vi "Write.vi"(8 "error in (no error)":errorcluster, 10 "Bytes":u8[](array[numeric]) format="%08b", 11 "Connection in":refnum<class "Connection.lvclass">) -> (0 "error out":errorcluster, 3 "Connection":refnum<class "Connection.lvclass">)   [LabVIEW 2013, in "MQTT_Connection.lvlib" / "Connection.lvclass"]
uses:
  Connection.lvclass
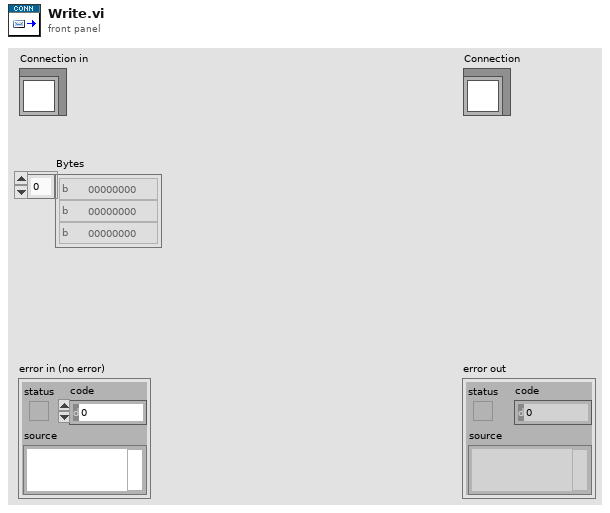
[diagram p1: front panel]
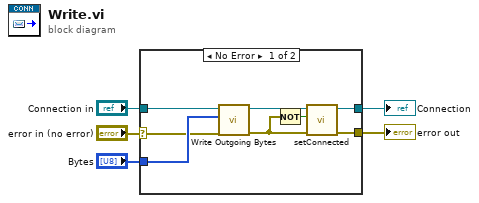
[diagram p0: block diagram]
diagram:
  n1 = case shown="No Error" "error in (no error)" {
    selector: "error in (no error)" -> [w11 w15]
    tunnel: [w8 w15] -> w4
    tunnel: [w9 w14] -> w2
    tunnel: "Connection in" -> [w13 w14]
    tunnel: "Bytes" -> [w12 _]
    frame No Error {
      n2 = call-dynamic "Write Outgoing Bytes.vi"("error in (no error)"=w11, "Bytes"=w12, "Connection in"=w13) -> ("error out"=w6:errorcluster, "Connection out"=w10:refnum<class "Connection.lvclass">)  [unwired: 7 in]
      n3 = Not(x=w6) -> (.not. x?=w7:bool)
      n4 = call "setConnected.vi"("error in (no error)"=w6, "connected"=w7, "Connection in"=w10) -> ("error out"=w8:errorcluster, "Connection out"=w9:refnum<class "Connection.lvclass">)  [unwired: 7 in]
    }
    frame Error {
    }
  }
  "error out" <- w4
  "Connection" <- w2
